vi "MandelbrotInner.vi"(5 "Numeric":cdb) -> (1 "Numeric 2":cdb)   [LabVIEW 2013]
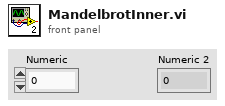
[diagram p1: front panel]
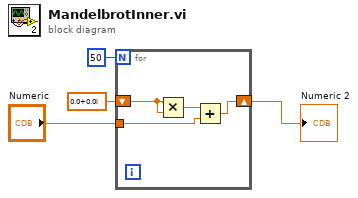
[diagram p0: block diagram]
diagram:
  n1 = for {
    N: 50 -> [_]
    shift-right: [w6] -> w2
    shift-left: cdb 0.0+0.0i -> [w8]
    tunnel: "Numeric" -> [w5]
    n2 = Multiply(x=w8, y=w8) -> (x*y=w7:cdb)
    n3 = Add(x=w7, y=w5) -> (x+y=w6:cdb)
  }
  "Numeric 2" <- w2
